vi "加标体积写入命令 (子VI).vi"(8 "错误输入（无错误）":errorcluster, 9 "values":u16[](array[numeric]), 10 "starting address":u16, 11 "Slave ID":u8=1) -> (0 "错误输出":errorcluster)   [LabVIEW 2016, in "质控单元.lvlib"]
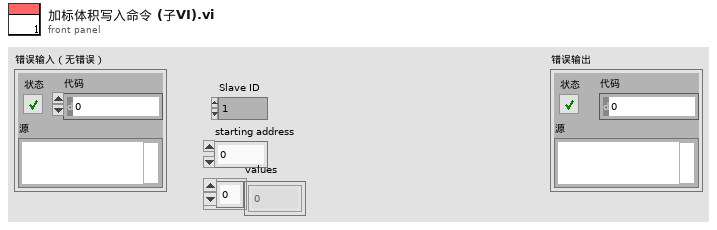
[diagram p1: front panel]
types:
  T1 = cluster{"starting address":u16, "values":u16[], "Slave ID":u8}
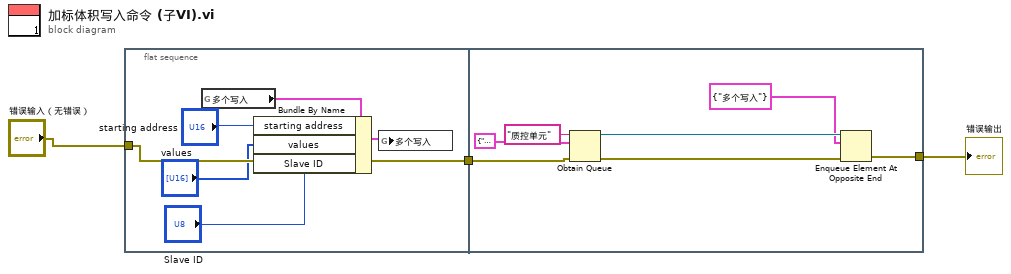
[diagram p0: block diagram]
diagram:
  n1 = flat-sequence {
    tunnel: "错误输入（无错误）" -> [w7]
    tunnel: [w7] -> w2
    tunnel: w2 -> [w11]
    tunnel: [w10] -> w1
    frame #0 {
      n2 = global read "质控内部交互全局.vi" "多个写入"() -> (w8:T1)
      n3 = Bundle By Name(cluster=w8, "starting address"="starting address", "values"="values", "Slave ID"="Slave ID") -> (w9:T1)
      n4 = global write "质控内部交互全局.vi" "多个写入"(w9) -> ()
    }
    frame #1 {
      n5 = Obtain Queue(name (unnamed)="质控单元" ("名称（未命名）"), element data type=cluster{"命令":string} {"命令"="启用模块"} ("元素"), error in (no error)=w11) -> (queue out=w14:refnum<queue>, error out=w13:errorcluster)  [unwired: 2 in, 1 out]
      n6 = Enqueue Element At Opposite End(queue=w14, element=cluster{"命令":string} {"命令"="多个写入"} ("元素"), error in (no error)=w13) -> (error out=w10:errorcluster)  [unwired: 1 in, 2 out]
    }
  }
  "错误输出" <- w1
